vi "Read Menu selections.vi"(8 "error in (no error)":errorcluster, 11 "Menu object parameters in":refnum<class "Menu object parameters.lvclass">) -> (0 "error out":errorcluster, 2 "Menu selections":string[](array[string]), 3 "Menu object parameters out":refnum<class "Menu object parameters.lvclass">)   [LabVIEW 2015, in "Menu object parameters.lvclass"]
uses:
  Menu object parameters.lvclass
  Menu object parameters.lvclass/Menu object parameters.ctl
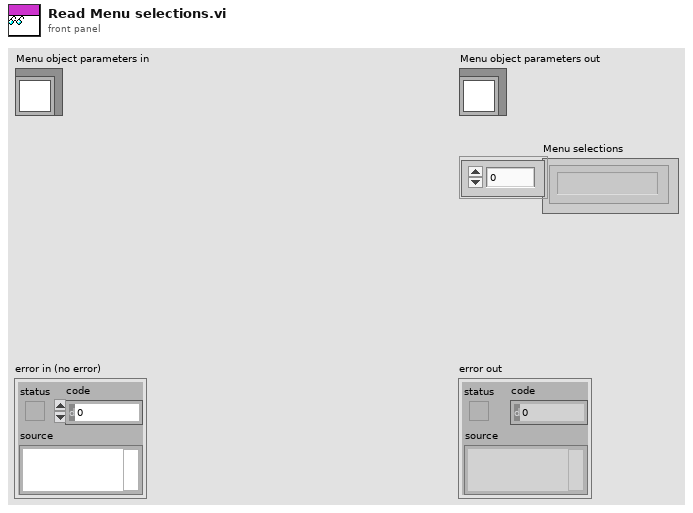
[diagram p1: front panel]
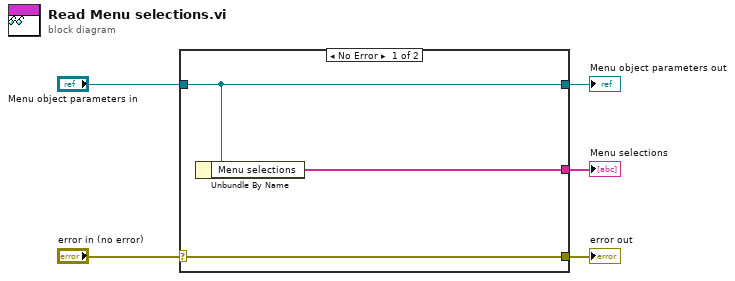
[diagram p0: block diagram]
diagram:
  n1 = case shown="No Error" "error in (no error)" {
    selector: "error in (no error)" -> [w8 w9]
    tunnel: [w8 w9] -> w4
    tunnel: [w7 w10] -> w2
    tunnel: "Menu object parameters in" -> [w7 w10]
    tunnel: [w6 _] -> w1
    frame No Error {
      n2 = Unbundle By Name(w7) -> ("Menu selections"=w6:string[])
    }
    frame Error {
    }
  }
  "error out" <- w4
  "Menu object parameters out" <- w2
  "Menu selections" <- w1
